vi "Queue_Week10.vi"() -> ()   [LabVIEW 2013]
panel:
  out "Waveform Chart":dbl(graph)
  in  "Max":dbl=25.0 format="%#_13g"
  in  "Min":dbl=15.0 format="%#_13g"
  in  "Max/Consumer":dbl=25.0 format="%#_13g"
  in  "Min/Consumer":dbl=15.0 format="%#_13g"
  out "Alarms\nConsumer":dbl
  out "Alarms":dbl
  out "Elements in Queue":i32
  out "Alarm Indicator 2":bool
  out "Alarm Indicator":bool
  in  "Stop":bool
  out "Temp. Values":dbl
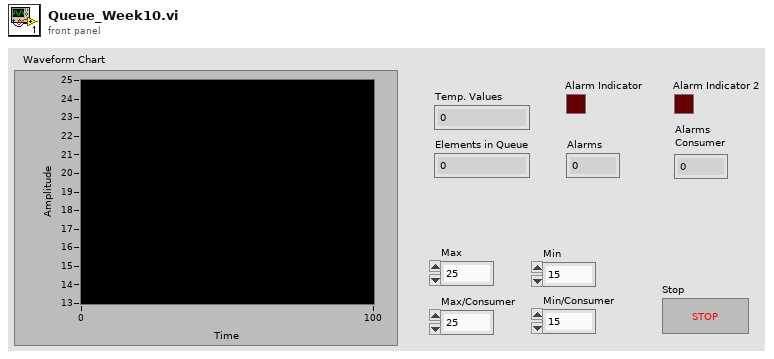
[diagram p1: front panel]
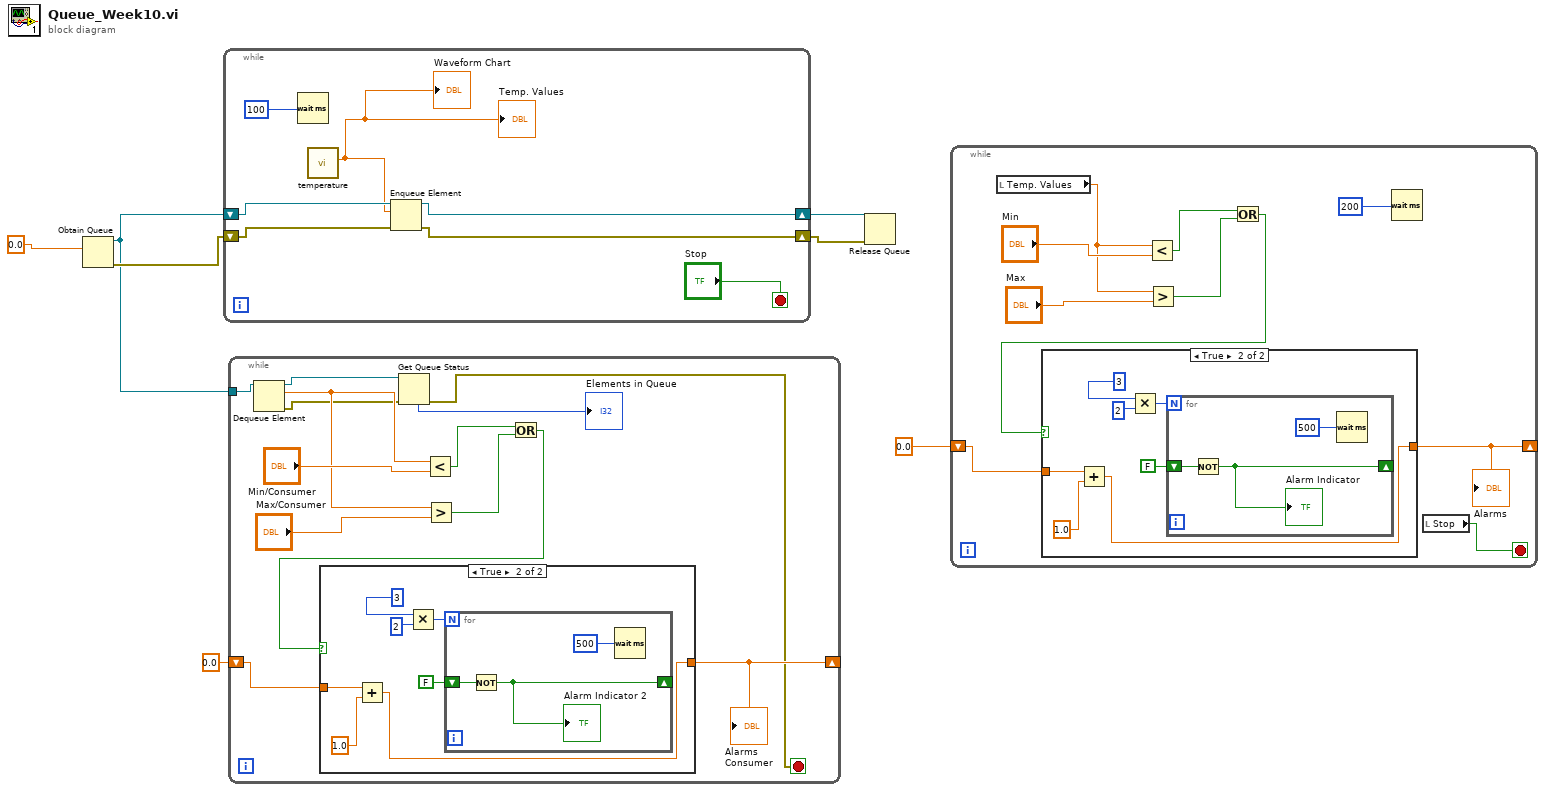
[diagram p0: block diagram]
diagram:
  n1 = Obtain Queue(element data type=0.0) -> (queue out=w1:refnum<queue>, error out=w6:errorcluster)  [unwired: 4 in, 1 out]
  n2 = while {
    shift-right: [w11] -> w5
    shift-left: w6 -> [w12]
    shift-right: [w9] -> w3
    shift-left: w1 -> [w10]
    stop <- "Stop" stop-if-true
    n3 = Wait (ms)(milliseconds to wait=100) -> ()  [unwired: 1 out]
    n4 = call "temperature.vi"() -> ("Temperature (C)"=w8:dbl)  [unwired: 10 in, 1 out]
    "Temp. Values" <- w8
    "Waveform Chart" <- w8
    n5 = Enqueue Element(queue=w10, element=w8, error in (no error)=w12) -> (queue out=w9:refnum<queue>, error out=w11:errorcluster)  [unwired: 1 in, 1 out]
  }
  n6 = while {
    shift-right: [w21] -> _
    shift-left: 0.0 -> [w22]
    tunnel: w1 -> [w20]
    stop <- w15 stop-if-true
    n7 = Dequeue Element(queue=w20) -> (queue out=w17:refnum<queue>, element=w19:dbl, error out=w18:errorcluster)  [unwired: 2 in, 1 out]
    n8 = Get Queue Status(queue=w17, error in (no error)=w18) -> (error out=w15:errorcluster, # elements in queue=→"Elements in Queue":i32)  [unwired: 1 in, 6 out]
    n9 = Less?(x=w19, y="Min/Consumer") -> (x < y?=w24:bool)
    n10 = Greater?(x=w19, y="Max/Consumer") -> (0:w25:bool)
    n11 = Or(x=w24, y=w25) -> (x .or. y?=w23:bool)
    n12 = case shown="True" w23 {
      tunnel: w22 -> [w28 w31]
      tunnel: [w28 w30] -> w21
      frame False {
      }
      frame True {
        n13 = Add(x=w31, y=1.0) -> (x+y=w30:dbl)
        n14 = Multiply(x=3, y=2) -> (x*y=w35:i32)
        n15 = for {
          N: w35 -> [_]
          shift-right: [w36] -> _
          shift-left: FALSE -> [w37]
          n16 = Not(x=w37) -> (.not. x?=w36:bool)
          "Alarm Indicator 2" <- w36
          n17 = Wait (ms)(milliseconds to wait=u32 500) -> ()  [unwired: 1 out]
        }
      }
    }
    "Alarms\nConsumer" <- w21
  }
  n18 = Release Queue(queue=w3, error in (no error)=w5) -> ()  [unwired: 1 in, 3 out]
  n19 = while {
    shift-right: [w39] -> _
    shift-left: 0.0 -> [w40]
    stop <- w41 stop-if-true
    n20 = local read "Temp. Values"() -> (w42:dbl)
    n21 = Less?(x=w42, y="Min") -> (x < y?=w45:bool)
    n22 = Greater?(x=w42, y="Max") -> (0:w46:bool)
    n23 = Or(x=w45, y=w46) -> (x .or. y?=w44:bool)
    n24 = case shown="True" w44 {
      tunnel: w40 -> [w49 w52]
      tunnel: [w49 w51] -> w39
      frame False {
      }
      frame True {
        n25 = Add(x=w52, y=1.0) -> (x+y=w51:dbl)
        n26 = Multiply(x=3, y=2) -> (x*y=w56:i32)
        n27 = for {
          N: w56 -> [_]
          shift-right: [w57] -> _
          shift-left: FALSE -> [w58]
          n28 = Not(x=w58) -> (.not. x?=w57:bool)
          "Alarm Indicator" <- w57
          n29 = Wait (ms)(milliseconds to wait=u32 500) -> ()  [unwired: 1 out]
        }
      }
    }
    "Alarms" <- w39
    n30 = Wait (ms)(milliseconds to wait=200) -> ()  [unwired: 1 out]
    n31 = local read "Stop"() -> (w41:bool)
  }
